vi "Database.vi"(8 "Options":T2(ring), 9 "Validity":dbl, 10 "Card Number":dbl, 11 "Card Holders Name":string) -> (1 "Search Results 1":T1(array[cluster]), 2 "Search Results 2":T1(array[cluster]), 3 "Search Results 3":T1(array[cluster]))   [LabVIEW 2014]
doc: "Database of employees. Employee details should be given as input .Search option is provided to search with respect to a particular element(Employee ID,Name,Validity)."
panel:
  in  "Reset":bool
  in  "Account Details":T1(array[cluster])
  # "Database for Employees"
  # "Database"
  # "Enter Database Details and Search for any element in the database."
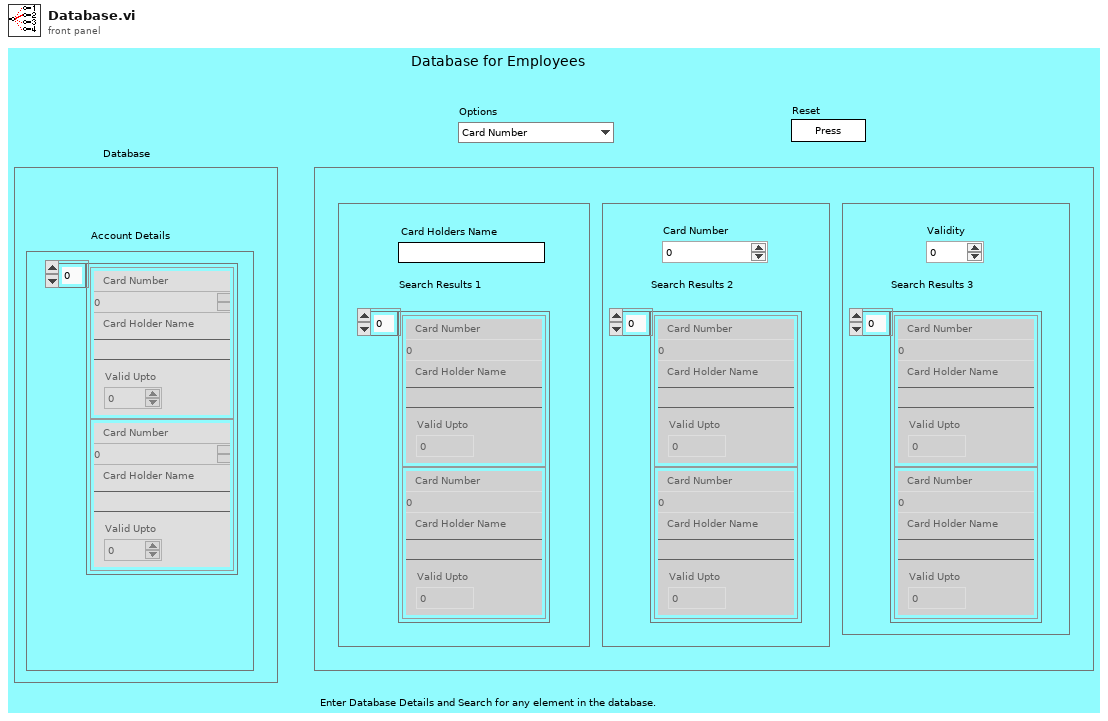
[diagram p1: front panel]
types:
  T1 = cluster{"Card Number":dbl, "Card Holder Name":string, "Valid Upto":dbl}[]
  T2 = enum16{"Card Number", "Card Holder Name", "Valid Upto"}
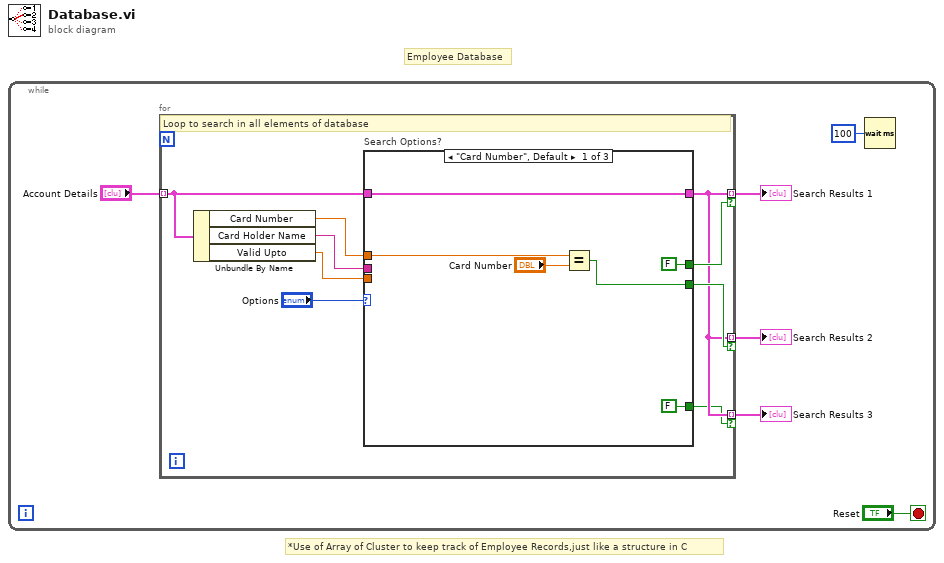
[diagram p0: block diagram]
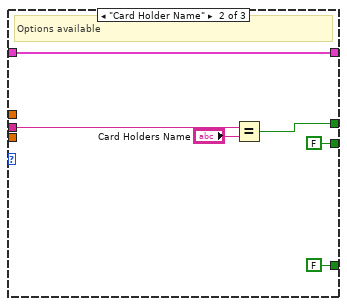
[diagram p2: hidden frame]
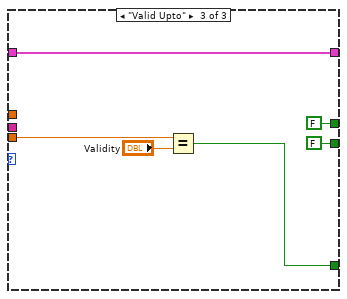
[diagram p3: hidden frame]
diagram:
  # "Employee Database"
  # "*Use of Array of Cluster to keep track of Employee Records,just like a structure in C"
  n1 = while {
    stop <- "Reset" stop-if-true
    n2 = for {
      tunnel: "Account Details" -> [w13] mode=indexing
      tunnel: [w8] -> w5 mode=indexing if=w10
      tunnel: [w8] -> w4 mode=indexing if=w9
      tunnel: [w8] -> w3 mode=indexing if=w7
      # "Loop to search in all elements of database"
      n3 = Unbundle By Name(w13) -> ("Card Number"=w14:dbl, "Card Holder Name"=w12:string, "Valid Upto"=w11:dbl)
      n4 = case "Search Options?" shown="\"Card Number\", Default" "Options" {
        tunnel: w14 -> [w20 _ _]
        tunnel: w13 -> [w17 w25 w31]
        tunnel: w12 -> [_ w27 _]
        tunnel: w11 -> [_ _ w33]
        tunnel: [w17 w25 w31] -> w8
        tunnel: [FALSE w24 FALSE] -> w10
        tunnel: [w19 FALSE FALSE] -> w9
        tunnel: [FALSE FALSE w30] -> w7
        frame "Card Number", Default {
          n5 = Equal?(x=w20, y="Card Number") -> (x = y?=w19:bool)
        }
        frame "Card Holder Name" {
          # "Options available"
          n6 = Equal?(x=w27, y="Card Holders Name") -> (x = y?=w24:bool)
        }
        frame "Valid Upto" {
          n7 = Equal?(x=w33, y="Validity") -> (x = y?=w30:bool)
        }
      }
    }
    "Search Results 1" <- w5
    "Search Results 2" <- w4
    "Search Results 3" <- w3
    n8 = Wait (ms)(milliseconds to wait=u32 100) -> ()  [unwired: 1 out]
  }
